vi "MT Compensate Sample Clock Frequency Error.vi"   [LabVIEW 2020, in "niDMT.lvlib"]
doc: "Estimates and corrects sample clock frequency offset, which is the difference between the sample clocks at the D/A converter of the transmitting DUT and digitizer. Use this VI before calling the Demodulation VIs."
uses:
  <vilib>/addons/Modulation/niDMT.lvlib
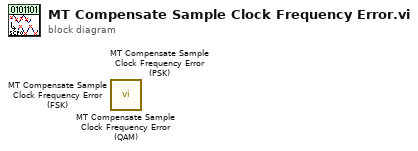
[diagram p0: block diagram]
diagram:
  n1 = call <vilib>:"MT Compensate Sample Clock Frequency Error (QAM).vi"() -> ()  [unwired: 13 in, 3 out]
  n2 = call <vilib>:"MT Compensate Sample Clock Frequency Error (PSK).vi"() -> ()  [unwired: 13 in, 3 out]
  n3 = call <vilib>:"MT Compensate Sample Clock Frequency Error (FSK).vi"() -> ()  [unwired: 13 in, 3 out]
